vi "HSOpMuxSingleSignal.vi"() -> ()   [LabVIEW 2013]
uses:
  Multiplexer_Opmux.lvclass
  <vilib>/Analysis/3filter.llb/Filter Passband Type.ctl
  <vilib>/measure/mamon.llb/Trigger Detection for 1 Channel.vi
  <vilib>/Analysis/3filter.llb/Butterworth Filter (DBL).vi
  OverallRoutines/HS3OverallRoutines.lvlib
  <vilib>/measure/NI_MAPro.lvlib
  <vilib>/Analysis/NI_AALBase.lvlib
panel:
  in  "Filter?":bool
  out "Cursors":i32[](array[numeric])
  out "lstTrgIdx":i32
  out "tmr":u32 caption="Elapsed for acq"
  in  "Run":bool
  out "Channels":refnum<vi>[](array[refnum])
  out "Ch8":dbl[](graph)
  out "Ch7":dbl[](graph)
  out "Ch6":dbl[](graph)
  out "Ch5":dbl[](graph)
  out "Ch4":dbl[](graph)
  out "Ch3":dbl[](graph)
  out "Ch2":dbl[](graph)
  out "Ch1":dbl[](graph)
  in  "Scan":bool
  in  "Set":bool
  in  "Length":dbl=1.0 caption="Length (us)" min=0.1 max=6.3 step=0.1
  in  "Voltage":dbl min=0.0 max=1023.0 step=1.0
  in  "Forward":u16[](array[numeric])
  in  "Signal Frequency":u32(ring)=10000000 items=["5Mhz"=5000000, "10Mhz"=10000000, "25Mhz"=25000000]
  in  "Shutdown":bool
  out "Acq":bool caption="Acquiring"
  out "SampleFrequency":dbl format="%#_8g"
  out "ChArray":dbl[](array[numeric])
  out "Serial":i32
  out "DllPath":path
  out "HandyScope":bool
  out "Multiplexer":bool
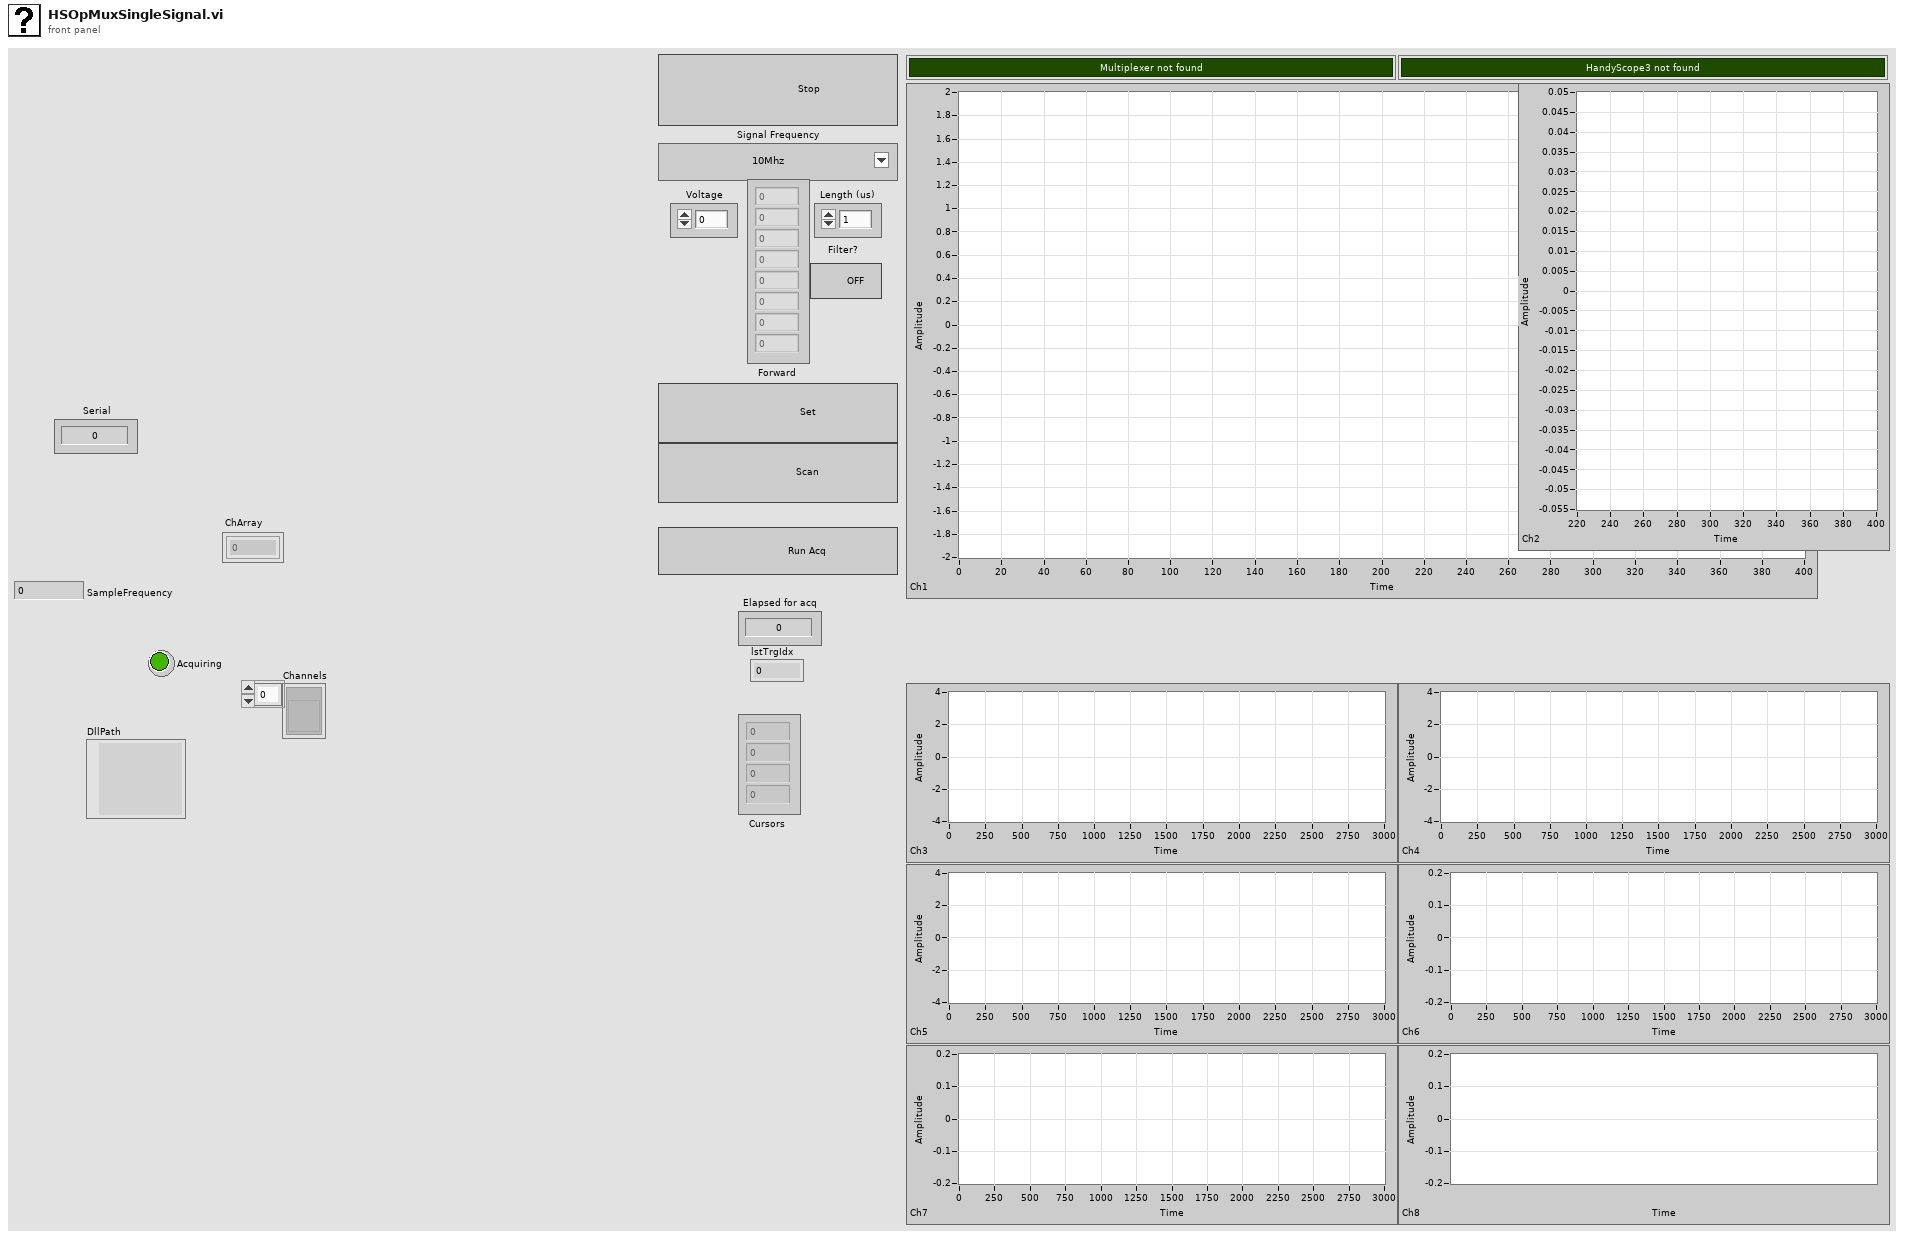
[diagram p1: front panel]
types:
  T1 = cluster{"trgSource":u16, "trgMode":u16, "trgLevel":dbl}
  T2 = typedef "NI_AALBase.lvlib/Filter Passband Type.ctl" = enum32{"Lowpass", "Highpass", "Bandpass", "Bandstop"}
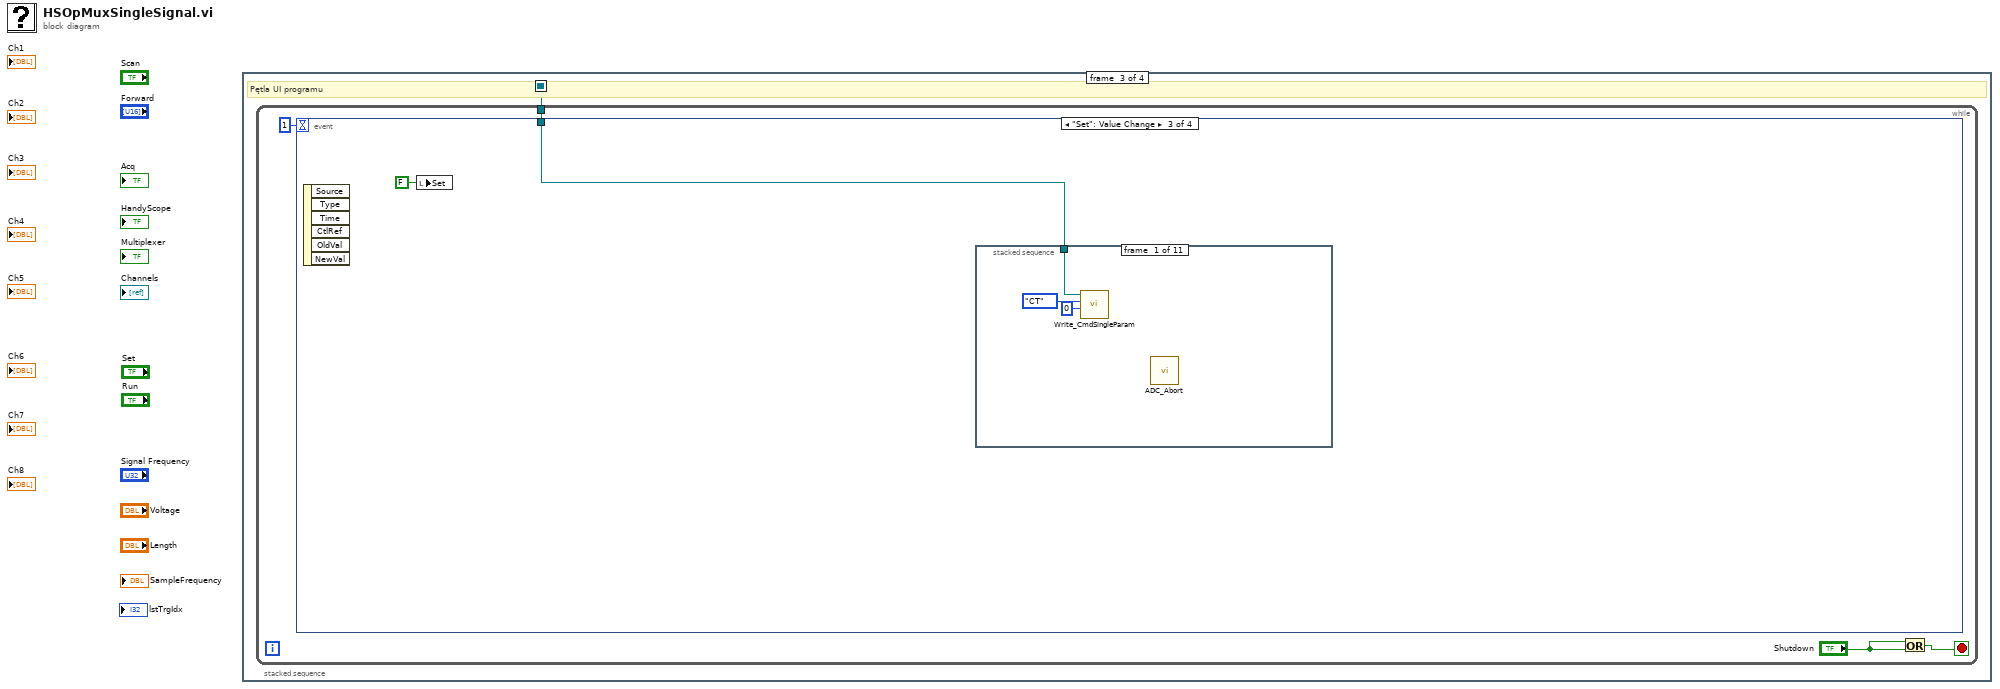
[diagram p0: block diagram]
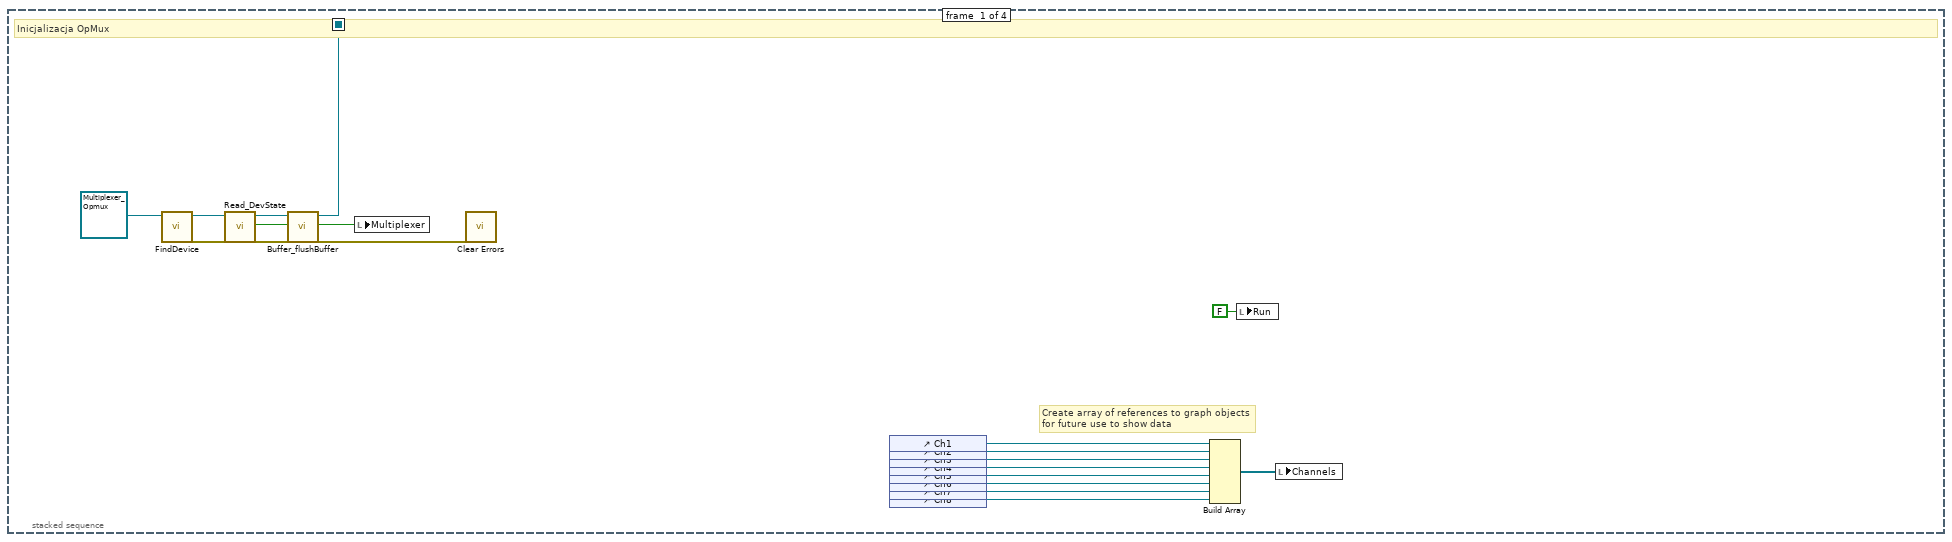
[diagram p2: hidden frame]
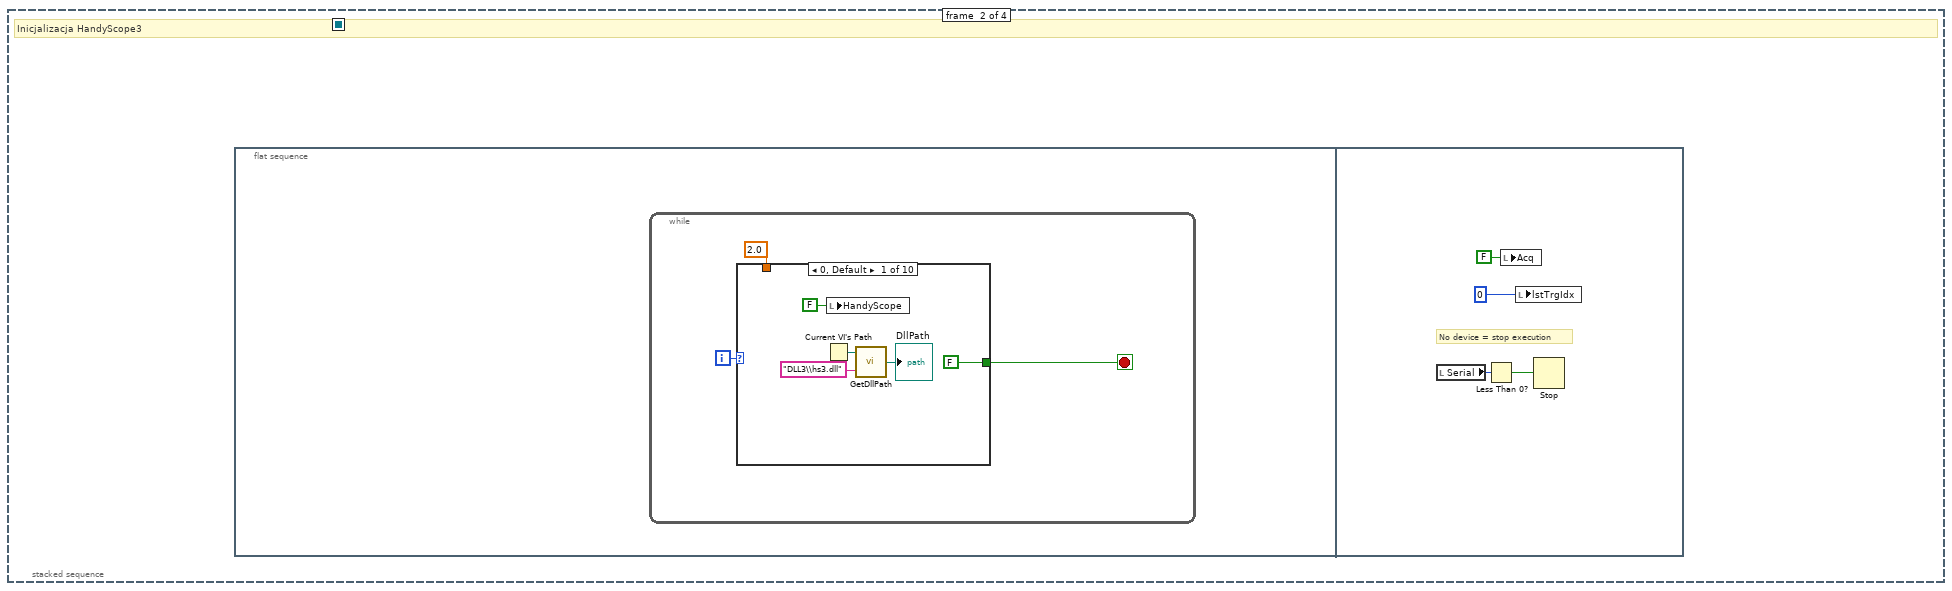
[diagram p3: hidden frame]
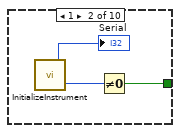
[diagram p4: hidden frame]
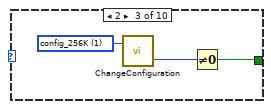
[diagram p5: hidden frame]
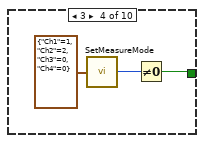
[diagram p6: hidden frame]
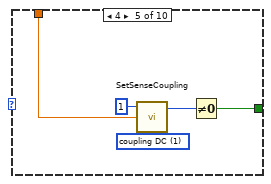
[diagram p7: hidden frame]
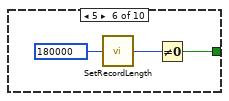
[diagram p8: hidden frame]
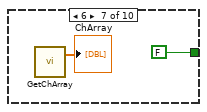
[diagram p9: hidden frame]
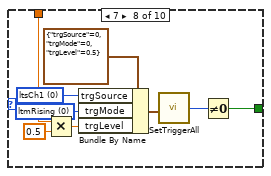
[diagram p10: hidden frame]
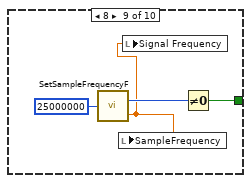
[diagram p11: hidden frame]
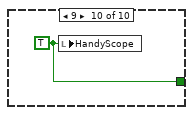
[diagram p12: hidden frame]
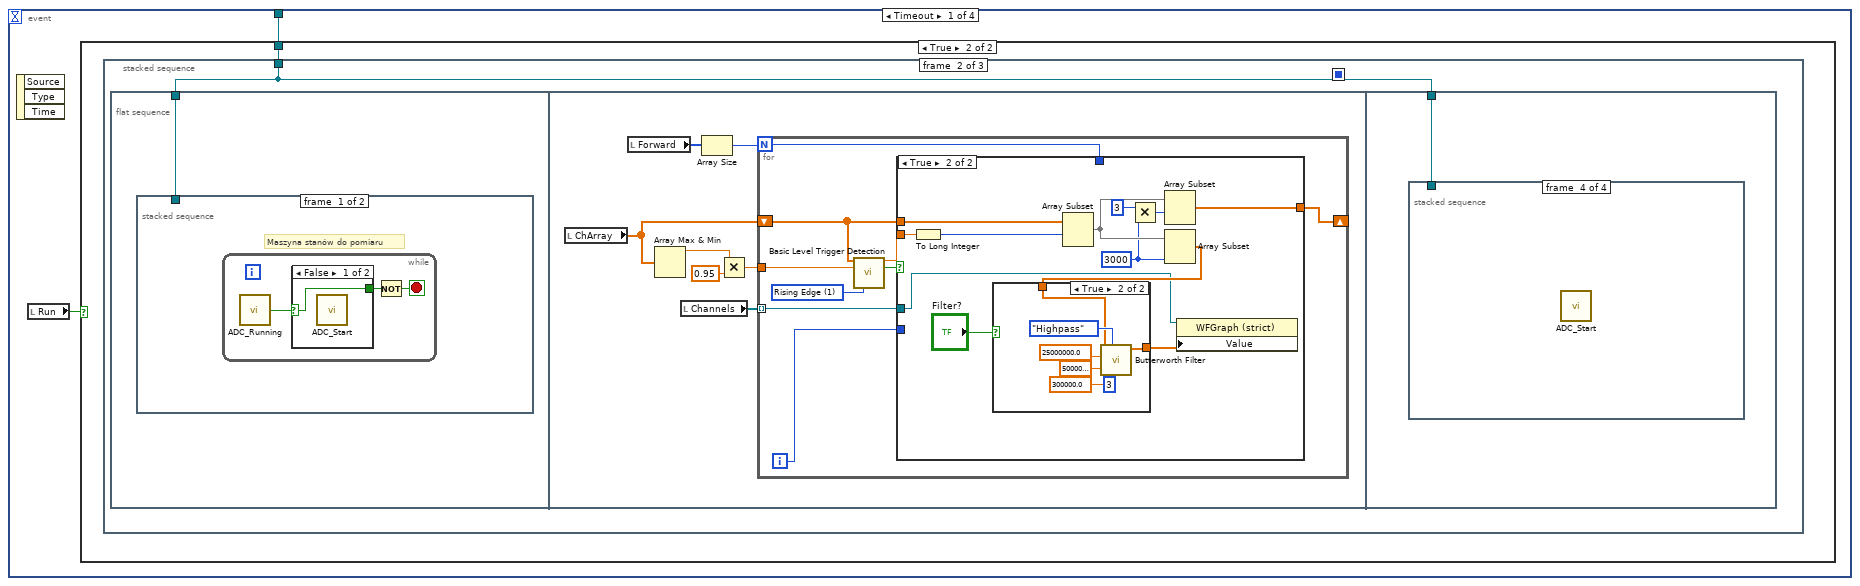
[diagram p13: hidden frame]
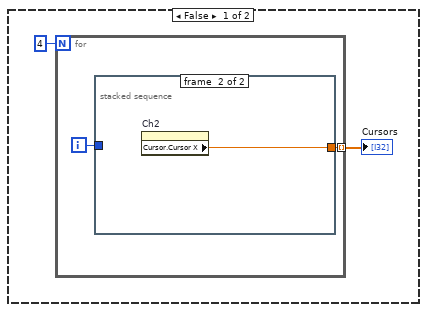
[diagram p14: hidden frame]
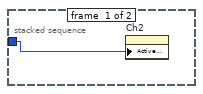
[diagram p15: hidden frame]
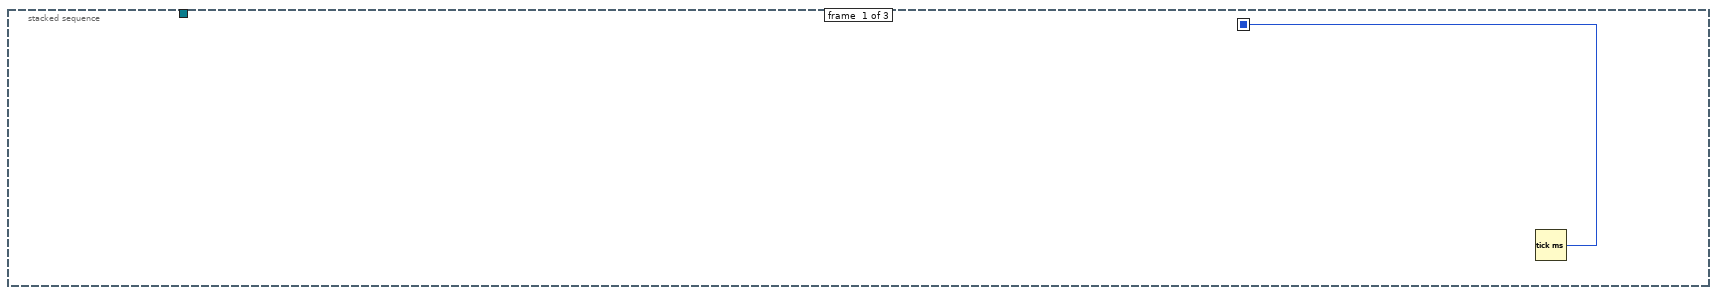
[diagram p16: hidden frame]
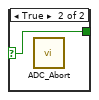
[diagram p17: hidden frame]
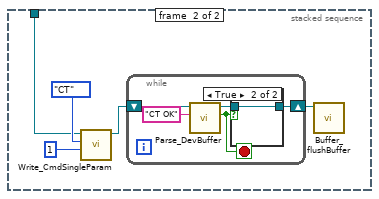
[diagram p18: hidden frame]
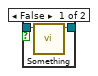
[diagram p19: hidden frame]
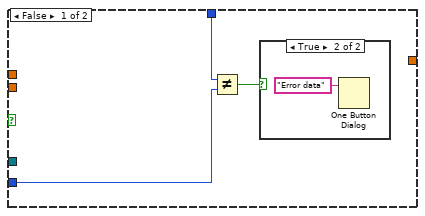
[diagram p20: hidden frame]
diagram:
  n1 = stacked-sequence {
    seq-local: [w1 _ _ _] -> [_ _ w64 _]
    frame #0 {
      # "Create array of references to graph objects\nfor future use to show data"
      # "Inicjalizacja OpMux"
      n2 = call-dynamic "FindDevice.vi"("Multiplexer_Opmux in"=refnum<class "Multiplexer_Opmux.lvclass"> refnum) -> ("error out"=w15:errorcluster, "Multiplexer_Opmux out"=w17:refnum<class "Multiplexer_Opmux.lvclass">)  [unwired: 8 in, 1 out]
      n3 = call-dynamic "Read_DevState.vi"("error in (no error)"=w15, "Multiplexer_Opmux in"=w17) -> ("error out"=w3:errorcluster, "DevState"=w16:bool, "Multiplexer_Opmux out"=w4:refnum<class "Multiplexer_Opmux.lvclass">)  [unwired: 7 in]
      n4 = call-dynamic "Buffer_flushBuffer.vi"("error in (no error)"=w3, "Multiplexer_Opmux in"=w4) -> ("error out"=w2:errorcluster, "Multiplexer_Opmux out"=w1:refnum<class "Multiplexer_Opmux.lvclass">)  [unwired: 8 in]
      n5 = local write "Multiplexer"(w16) -> ()
      n6 = call <vilib>:"Clear Errors.vi"("error in (no error)"=w2) -> ()  [unwired: 6 in, 1 out]
      n7 = control-ref of="Ch1"() -> (w14:refnum<vi>)
      n8 = control-ref of="Ch2"() -> (w13:refnum<vi>)
      n9 = control-ref of="Ch3"() -> (w12:refnum<vi>)
      n10 = control-ref of="Ch4"() -> (w11:refnum<vi>)
      n11 = control-ref of="Ch5"() -> (w10:refnum<vi>)
      n12 = control-ref of="Ch6"() -> (w9:refnum<vi>)
      n13 = control-ref of="Ch7"() -> (w8:refnum<vi>)
      n14 = control-ref of="Ch8"() -> (w7:refnum<vi>)
      n15 = Build Array(w14, w13, w12, w11, w10, w9, w8, w7) -> (w6:refnum<vi>[])
      n16 = local write "Run"(FALSE ("Run")) -> ()
      n17 = local write "Channels"(w6) -> ()
    }
    frame #1 {
      # "Inicjalizacja HandyScope3"
      n18 = flat-sequence {
        frame #0 {
          n19 = while {
            i -> [w21]
            stop <- w20 stop-if-true
            w19 = 2.0 items=["0,2"=0.2, "0,8"=0.8, "2"=2.0, "4"=4.0, "20"=20.0, "40"=40.0, "80"=80.0] ("chSense")
            n20 = case shown="0, Default" w21 {
              tunnel: [FALSE w27 w32 w34 w37 w42 FALSE w53 w58 w59] -> w20
              tunnel: w19 -> [_ _ _ _ w36 _ _ w49 _ _]
              frame 0, Default {
                n21 = Current VI's Path() -> (path=w24:path)
                n22 = local write "HandyScope"(FALSE ("HandyScope")) -> ()
                n23 = call "GetDllPath.vi"("DllName"="DLL3\\hs3.dll", "path"=w24) -> ("DllPath"=→"DllPath":path)
              }
              frame 1 {
                n24 = call "InitializeInstrument.vi"() -> ("ErrorCode"=w28:i16, "Serial"=→"Serial":i32)
                n25 = Not Equal To 0?(x=w28) -> (x != 0?=w27:bool)
              }
              frame 2 {
                w30 = u16 1 items=["config_Normal", "config_256K", "config_512K"] ("config")
                n26 = call "ChangeConfiguration.vi"("config"=w30) -> ("ErrorCode"=w31:i16)
                n27 = Not Equal To 0?(x=w31) -> (x != 0?=w32:bool)
              }
              frame 3 {
                n28 = call "SetMeasureMode.vi"("oModeStack"=cluster{"Ch1":u8, "Ch2":u8, "Ch3":u8, "Ch4":u8} {"Ch1"=1, "Ch2"=2, "Ch3"=0, "Ch4"=0}) -> ("ErrorCode"=w33:i16)
                n29 = Not Equal To 0?(x=w33) -> (x != 0?=w34:bool)
              }
              frame 4 {
                w40 = 1 items=["coupling AC", "coupling DC"] ("chCoupling")
                n30 = call "SetSenseCoupling.vi"("chCoupling"=w40, "chSense"=w36, "chSet"=1) -> ("ErrorCode"=w38:i16)  [unwired: 1 out]
                n31 = Not Equal To 0?(x=w38) -> (x != 0?=w37:bool)
              }
              frame 5 {
                w43 = u32 180000 items=["100"=100, "250"=250, "500"=500, "1000"=1000, "2500"=2500, "5000"=5000, "10000"=10000, "25000"=25000, "50000"=50000, "100000"=100000, "131000"=131000, "180000"=180000, "256000"=256000] ("RecordLength")
                n32 = call "SetRecordLength.vi"("RecordLength"=w43) -> ("ErrorCode"=w41:i16)
                n33 = Not Equal To 0?(x=w41) -> (x != 0?=w42:bool)
              }
              frame 6 {
                n34 = call "GetChArray.vi"() -> ("ChArray"=→"ChArray":dbl[])  [unwired: 1 out]
              }
              frame 7 {
                w46 = u16 0 items=["ltmRising", "ltmFalling", "ltmInWindow", "ltmOutWindow", "ltmTVLine", "ltmTVFieldOdd", "ltmTVFieldEven"] ("trgMode")
                w47 = u16 0 items=["ltsCh1"=0, "ltsCh2"=1, "ltsExternal"=4, "ltsAnalogExt"=5, "ltsAnd"=6, "ltsOr"=7, "ltsXor"=8, "ltsNoTrig"=9, "notUsed"=10, "ltsPxiExt"=11, "ltsGenStart"=12, "ltsGenStop"=13, "ltsGenNew"=14] ("trgSource")
                n35 = Multiply(x=w49, y=0.5) -> (x*y=w50:dbl)
                n36 = Bundle By Name(cluster=T1 {"trgSource"=0, "trgMode"=0, "trgLevel"=0.5} ("TriggerSettings"), "trgSource"=w47, "trgMode"=w46, "trgLevel"=w50) -> (w51:T1)
                n37 = call "SetTriggerAll.vi"("TriggerSettings"=w51) -> ("ErrorCode"=w54:i32)
                n38 = Not Equal To 0?(x=w54) -> (x != 0?=w53:bool)
              }
              frame 8 {
                n39 = call "SetSampleFrequencyF.vi"("Numeric Control"=u32 25000000) -> ("ErrorCode"=w57:i16, "oFreq_Set"=w56:dbl)
                n40 = local write "SampleFrequency"(w56) -> ()
                n41 = local write "Signal Frequency"(w56) -> ()
                n42 = Not Equal To 0?(x=w57) -> (x != 0?=w58:bool)
              }
              frame 9 {
                w59 = TRUE ("HandyScope")
                n43 = local write "HandyScope"(w59) -> ()
              }
            }
          }
        }
        frame #1 {
          # "No device = stop execution"
          n44 = local read "Serial"() -> (w63:i32)
          n45 = Less Than 0?(x=w63) -> (x < 0?=w62:bool)
          n46 = local write "Acq"(FALSE ("Acq")) -> ()
          n47 = local write "lstTrgIdx"(0 ("LastTriggerIndex")) -> ()
          n48 = Stop(stop? (T)=w62) -> ()
        }
      }
    }
    frame #2 {
      # "Pętla UI programu"
      n49 = while {
        tunnel: w64 -> [w65]
        stop <- w67 stop-if-true
        n50 = event shown="[2] \"Set\": Value Change" {
          selector: _ -> [_ _ _ _]
          dyn-events: _ -> [_ _ _ _]
          timeout: 1 -> [_ _ _ _]
          tunnel: w65 -> [w70 _ w161 _]
          event Timeout {
            n51 = event-data() -> ()  [unwired: 1 in, 3 out]
            n52 = local read "Run"() -> (w69:bool)
            n53 = case shown="True" w69 {
              tunnel: w70 -> [_ w77]
              frame False {
                n54 = for {
                  N: 4 -> [_]
                  tunnel: [w73] -> w71 mode=indexing
                  i -> [w74]
                  n55 = stacked-sequence {
                    tunnel: w74 -> [w75 _]
                    tunnel: [_ w76] -> w73
                    frame #0 {
                      n56 = property on="Ch2" class="WFGraph (strict)"("Active Cursor"=w75) -> ()  [unwired: 2 in, 2 out]
                    }
                    frame #1 {
                      n57 = property on="Ch2" class="WFGraph (strict)"() -> ("Cursor.Cursor X"=w76:dbl)  [unwired: 2 in, 2 out]
                    }
                  }
                }
                "Cursors" <- w71
              }
              frame True {
                n58 = stacked-sequence {
                  seq-local: [w78 _ _] -> [_ _ w158]
                  tunnel: w77 -> [_ w79 _]
                  frame #0 {
                    n59 = Tick Count (ms)() -> (millisecond timer value=w78:u32)
                  }
                  frame #1 {
                    n60 = flat-sequence {
                      tunnel: w79 -> [w80]
                      tunnel: w79 -> [w139]
                      frame #0 {
                        n61 = stacked-sequence {
                          tunnel: w80 -> [_ w86]
                          frame #0 {
                            # "Maszyna stanów do pomiaru"
                            n62 = while {
                              stop <- w82 stop-if-true
                              n63 = call "ADC_Running.vi"() -> ("Measuring"=w83:bool)
                              n64 = case shown="False" w83 {
                                selector: w83 -> [w84 w85]
                                tunnel: [w84 w85] -> w81
                                frame False {
                                n65 = call "ADC_Start.vi"() -> ()  [unwired: 1 out]
                                }
                                frame True {
                                n66 = call "ADC_Abort.vi"() -> ()  [unwired: 1 out]
                                }
                              }
                              n67 = Not(x=w81) -> (.not. x?=w82:bool)
                            }
                          }
                          frame #1 {
                            n68 = call-dynamic "Write_CmdSingleParam.vi"("Param"=1, "Command"=enum16{"SA", "GT", "SI", "SL", "ST", "CT"}."CT", "Multiplexer_Opmux in"=w86) -> ("Multiplexer_Opmux out"=w88:refnum<class "Multiplexer_Opmux.lvclass">)  [unwired: 7 in, 1 out]
                            n69 = while {
                              shift-right: [w92] -> w87
                              shift-left: w88 -> [w91]
                              stop <- w94 stop-if-true
                              n70 = call-dynamic "Parse_DevBuffer.vi"("searchFor"="CT OK", "Multiplexer_Opmux in"=w91) -> ("Found"=w94:bool, "Multiplexer_Opmux out"=w95:refnum<class "Multiplexer_Opmux.lvclass">)  [unwired: 7 in, 1 out]
                              n71 = case shown="True" w94 {
                                tunnel: w95 -> [w97 w98]
                                tunnel: [w96 w98] -> w92
                                frame False {
                                n72 = call-dynamic "Something.vi"("Multiplexer_Opmux in"=w97) -> ("Multiplexer_Opmux out"=w96:refnum<class "Multiplexer_Opmux.lvclass">)  [unwired: 9 in, 1 out]
                                }
                                frame True {
                                }
                              }
                            }
                            n73 = call-dynamic "Buffer_flushBuffer.vi"("Multiplexer_Opmux in"=w87) -> ()  [unwired: 9 in, 2 out]
                          }
                        }
                      }
                      frame #1 {
                        n74 = local read "ChArray"() -> (w99:dbl[])
                        n75 = local read "Forward"() -> (w101:u16[])
                        n76 = Array Max & Min(array=w99) -> (max value=w104:dbl)  [unwired: 3 out]
                        n77 = local read "Channels"() -> (w102:refnum<vi>[])
                        n78 = Array Size(array=w101) -> (size(s)=w100:i32)
                        n79 = Multiply(x=w104, y=0.95) -> (x*y=w103:dbl)
                        n80 = for {
                          N: w100 -> [w107]
                          shift-right: [w111] -> _
                          shift-left: w99 -> [w106]
                          tunnel: w103 -> [w110]
                          tunnel: w102 -> [w108] mode=indexing
                          i -> [w109]
                          w114 = u16 1 items=["Falling Edge", "Rising Edge"] ("trigger slope")
                          n81 = call-poly <vilib>:"Basic Level Trigger Detection.vi"("signal in"=w106, "level"=w110, "trigger slope"=w114) -> ("trigger location"=w112:dbl, "trigger detected?"=w113:bool)  [unwired: 10 in, 1 out]
                          n82 = case shown="True" w113 {
                            tunnel: w106 -> [_ w130]
                            tunnel: w112 -> [_ w129]
                            tunnel: [_ w126] -> w111
                            tunnel: w109 -> [w117 _]
                            tunnel: w108 -> [_ w119]
                            tunnel: w107 -> [w115 _]
                            frame False {
                              n83 = Not Equal?(x=w115, y=w117) -> (x != y?=w116:bool)
                              n84 = case shown="True" w116 {
                                frame False {
                                }
                                frame True {
                                n85 = One Button Dialog(message="Error data") -> ()  [unwired: 1 in, 1 out]
                                }
                              }
                            }
                            frame True {
                              w124 = 3000 ("length")
                              n86 = To Long Integer(number=w129) -> (32bit integer=w128:i32)
                              n87 = Array Subset(array=w130, index=w128) -> (w127:dbl[])  [unwired: 1 in]
                              n88 = Multiply(x=3, y=w124) -> (x*y=w125:i32)
                              n89 = Array Subset(array=w127, index=w125) -> (w126:dbl[])  [unwired: 1 in]
                              n90 = Array Subset(array=w127, length=w124) -> (w122:dbl[])  [unwired: 1 in]
                              n91 = case shown="True" "Filter?" {
                                tunnel: w122 -> [w131 w132]
                                tunnel: [w131 w133] -> w121
                                frame False {
                                }
                                frame True {
                                n92 = call-poly <vilib>:"Butterworth Filter.vi"("order"=3, "filter type"=Filter_Passband_Type."Highpass", "low cutoff freq: fl"=300000.0, "high cutoff freq: fh"=5000000.0, "sampling freq: fs"=25000000.0, "X"=w132) -> ("Filtered X"=w133:dbl[])  [unwired: 2 in, 1 out]
                                }
                              }
                              n93 = property class="WFGraph (strict)"(reference=w119, "Value"=w121) -> ()  [unwired: 1 in, 2 out]
                            }
                          }
                        }
                      }
                      frame #2 {
                        n94 = stacked-sequence {
                          tunnel: w139 -> [_ _ w144 _]
                          frame #0 {
                            n95 = while {
                              stop <- w141 stop-if-true
                              n96 = call "ADC_Ready.vi"() -> ("Ready"=w141:bool)
                            }
                            n97 = local write "lstTrgIdx"(0 ("LastTriggerIndex")) -> ()
                          }
                          frame #1 {
                            n98 = local read "ChArray"() -> (w143:dbl[])
                            n99 = call "GetDataVoltChAdvanced.vi"("chData"=w143) -> ("chOutData"=w142:dbl[])  [unwired: 1 out]
                            n100 = local write "ChArray"(w142) -> ()
                          }
                          frame #2 {
                            n101 = call-dynamic "Write_CmdSingleParam.vi"("Param"=0, "Command"=enum16{"SA", "GT", "SI", "SL", "ST", "CT"}."CT", "Multiplexer_Opmux in"=w144) -> ("Multiplexer_Opmux out"=w146:refnum<class "Multiplexer_Opmux.lvclass">)  [unwired: 7 in, 1 out]
                            n102 = while {
                              shift-right: [w150] -> w145
                              shift-left: w146 -> [w149]
                              stop <- w152 stop-if-true
                              n103 = call-dynamic "Parse_DevBuffer.vi"("searchFor"="CT OK", "Multiplexer_Opmux in"=w149) -> ("Found"=w152:bool, "Multiplexer_Opmux out"=w153:refnum<class "Multiplexer_Opmux.lvclass">)  [unwired: 7 in, 1 out]
                              n104 = case shown="True" w152 {
                                tunnel: w153 -> [w155 w156]
                                tunnel: [w154 w156] -> w150
                                frame False {
                                n105 = call-dynamic "Something.vi"("Multiplexer_Opmux in"=w155) -> ("Multiplexer_Opmux out"=w154:refnum<class "Multiplexer_Opmux.lvclass">)  [unwired: 9 in, 1 out]
                                }
                                frame True {
                                }
                              }
                            }
                            n106 = call-dynamic "Buffer_flushBuffer.vi"("Multiplexer_Opmux in"=w145) -> ()  [unwired: 9 in, 2 out]
                          }
                          frame #3 {
                            n107 = call "ADC_Start.vi"() -> ()  [unwired: 1 out]
                          }
                        }
                      }
                    }
                  }
                  frame #2 {
                    n108 = Tick Count (ms)() -> (millisecond timer value=w159:u32)
                    n109 = Subtract(x=w159, y=w158) -> (x-y=→"tmr":u32)
                  }
                }
              }
            }
          }
          event "Scan": Value Change {
            n110 = event-data() -> ()  [unwired: 1 in, 6 out]
          }
          event "Set": Value Change {
            n111 = event-data() -> ()  [unwired: 1 in, 6 out]
            n112 = local write "Set"(FALSE ("Set")) -> ()
            n113 = stacked-sequence {
              tunnel: w161 -> [w164 _ w167 _ w170 _ w176 _ w180 _ w182]
              frame #0 {
                n114 = call-dynamic "Write_CmdSingleParam.vi"("Param"=0, "Command"=enum16{"SA", "GT", "SI", "SL", "ST", "CT"}."CT", "Multiplexer_Opmux in"=w164) -> ()  [unwired: 7 in, 2 out]
                n115 = call "ADC_Abort.vi"() -> ()  [unwired: 1 out]
              }
              frame #1 {
                n116 = Wait (ms)(milliseconds to wait=u32 50) -> ()  [unwired: 1 out]
              }
              frame #2 {
                n117 = local read "Forward"() -> (w166:u16[])
                n118 = call-dynamic "Write_CmdMultipleParam.vi"("Command"=enum16{"ST"}."ST", "Table2"=w166, "Table1"=w166, "Multiplexer_Opmux in"=w167) -> ()  [unwired: 6 in, 2 out]
              }
              frame #3 {
                n119 = Wait (ms)(milliseconds to wait=u32 50) -> ()  [unwired: 1 out]
              }
              frame #4 {
                n120 = local read "Length"() -> (w172:dbl)
                n121 = Multiply(x=w172, y=10.0) -> (x*y=w173:dbl)
                n122 = call-dynamic "Write_CmdSingleParam.vi"("Param"=w173, "Command"=enum16{"SA", "GT", "SI", "SL", "ST", "CT"}."SL", "Multiplexer_Opmux in"=w170) -> ()  [unwired: 7 in, 2 out]
              }
              frame #5 {
                n123 = Wait (ms)(milliseconds to wait=u32 50) -> ()  [unwired: 1 out]
              }
              frame #6 {
                n124 = local read "Voltage"() -> (w178:dbl)
                n125 = call-dynamic "Write_CmdSingleParam.vi"("Param"=w178, "Command"=enum16{"SA", "GT", "SI", "SL", "ST", "CT"}."SI", "Multiplexer_Opmux in"=w176) -> ()  [unwired: 7 in, 2 out]
              }
              frame #7 {
                n126 = Wait (ms)(milliseconds to wait=u32 50) -> ()  [unwired: 1 out]
              }
              frame #8 {
                n127 = call-dynamic "Buffer_flushBuffer.vi"("Multiplexer_Opmux in"=w180) -> ()  [unwired: 9 in, 2 out]
              }
              frame #9 {
                n128 = Wait (ms)(milliseconds to wait=u32 25) -> ()  [unwired: 1 out]
              }
              frame #10 {
                n129 = local write "Run"(TRUE ("Run")) -> ()
                n130 = call-dynamic "Write_CmdSingleParam.vi"("Param"=1, "Command"=enum16{"SA", "GT", "SI", "SL", "ST", "CT"}."CT", "Multiplexer_Opmux in"=w182) -> ()  [unwired: 7 in, 2 out]
              }
            }
          }
          event "Signal Frequency": Value Change {
            n131 = event-data() -> ("NewVal"=w186:u32)  [unwired: 1 in, 5 out]
            n132 = stacked-sequence {
              tunnel: w186 -> [w190 _]
              frame #0 {
                n133 = call "SetSampleFrequencyF.vi"("Numeric Control"=w190) -> ("ErrorCode"=w189:i16, "oFreq_Set"=w188:dbl)
                n134 = case shown="True" FALSE {
                  tunnel: w188 -> [_ w194]
                  frame False {
                  }
                  frame True {
                    # "Do 100us sygnał zmieniamy automatycznie"
                    n135 = Multiply(x=w194, y=0.0008) -> (x*y=w192:dbl)
                    n136 = To Unsigned Long Integer(number=w192) -> (unsigned 32bit integer=w193:u32)
                    n137 = call "SetRecordLength.vi"("RecordLength"=w193) -> ()  [unwired: 1 out]
                  }
                }
                n138 = local write "SampleFrequency"(w188) -> ()
                n139 = call "Error Converter (ErrCode or Status).vi"("error code"=w189) -> ()  [unwired: 10 in, 1 out]
              }
              frame #1 {
              }
            }
          }
        }
        n140 = Or(x="Shutdown", y="Shutdown") -> (x .or. y?=w67:bool)
      }
    }
    frame #3 {
      # "Rozłączenie urządzeń po zakończeniu działania programu"
    }
  }
